vi "ReservationMemory_CopyDataToGPU.vi"(0 "Array Src In Host":u8[](array[numeric]), 3 "Width":i32, 4 "Height":i32, 5 "Error In LabVIEW":errorcluster) -> (18 "Error OUT Toolkit":i32, 19 "Error Out LabVIEW":errorcluster)   [LabVIEW 2018]
doc: "It reserves in GPU memory two spaces for 1D Arrays U8 to perform operations inside it and copy one of them in GPU memory to work with that.\n\nIt is the initial VI of the DLL, this should pass the variable error to VI processing algorithm."
uses:
  dll/LibreriaAutis_3.dll
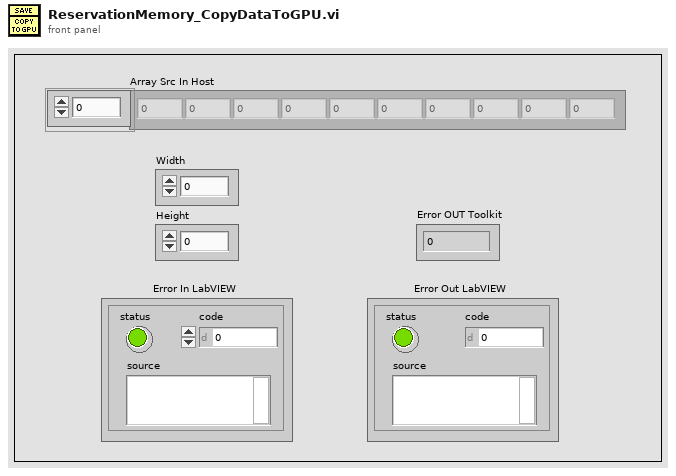
[diagram p1: front panel]
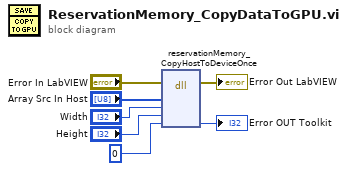
[diagram p0: block diagram]
diagram:
  n1 = dll-call lib="C:/Users/AUTIS/Desktop/LibreriaAUTIS/LabVIEW/dll/LibreriaAutis_3.dll" fn="reservationMemory_CopyHostToDeviceOnce"(error in="Error In LabVIEW", "src"="Array Src In Host", "w"="Width", "h"="Height", "error"=0) -> (error out=→"Error Out LabVIEW":errorcluster, "error"=→"Error OUT Toolkit":i32)  [unwired: 6 in, 1 out]
